vi "Generate Test Images.vi"() -> (0 "error out":errorcluster, 1 "queue out":refnum<queue>)   [LabVIEW 2018, in "Assembly Line Input.lvclass"]
doc: "Generate 50 test images of each type of board, with randomized failures."
uses:
  Assembly Line Input.lvclass
  Common/Board Type Enum.ctl
  Common/Board Image.ctl
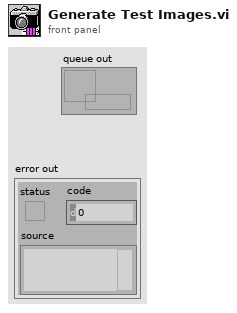
[diagram p1: front panel]
types:
  T1 = typedef "Board Type Enum.ctl" = enum16{"Basic DAQ Board", "Elite DAQ Board", "GPIB Board"}
  T2 = typedef "Board Image.ctl" = picture
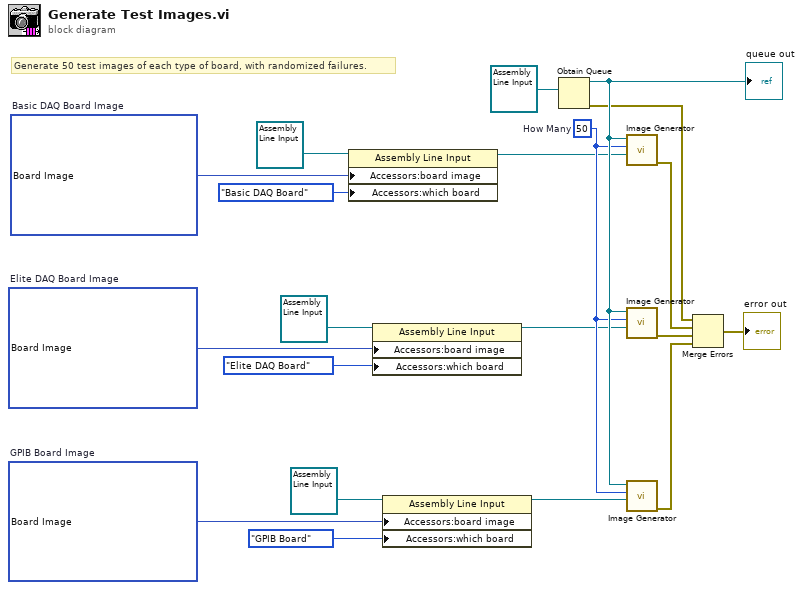
[diagram p0: block diagram]
diagram:
  w1 = T2 bytes[67710]  # GPIB Board Image
  w6 = T2 bytes[67710]  # Elite DAQ Board Image
  w11 = T2 bytes[67710]  # Basic DAQ Board Image
  w19 = 50  # How Many
  # "Generate 50 test images of each type of board, with randomized failures."
  n1 = property class="Assembly Line Input"(reference=refnum<class "Assembly Line Input.lvclass"> refnum ("Assembly Line Input"), "Accessors:board image"=w11, "Accessors:which board"=Board_Type_Enum."Basic DAQ Board" ("which board")) -> (reference out=w9:refnum<class "Assembly Line Input.lvclass">)  [unwired: 1 in, 1 out]
  n2 = property class="Assembly Line Input"(reference=refnum<class "Assembly Line Input.lvclass"> refnum ("Assembly Line Input"), "Accessors:board image"=w6, "Accessors:which board"=Board_Type_Enum."Elite DAQ Board" ("which board")) -> (reference out=w4:refnum<class "Assembly Line Input.lvclass">)  [unwired: 1 in, 1 out]
  n3 = property class="Assembly Line Input"(reference=refnum<class "Assembly Line Input.lvclass"> refnum ("Assembly Line Input"), "Accessors:board image"=w1, "Accessors:which board"=Board_Type_Enum."GPIB Board" ("which board")) -> (reference out=w2:refnum<class "Assembly Line Input.lvclass">)  [unwired: 1 in, 1 out]
  n4 = Obtain Queue(element data type=refnum<class "Assembly Line Input.lvclass"> refnum ("Assembly Line Input")) -> (queue out=w20:refnum<queue>, error out=w14:errorcluster)  [unwired: 4 in, 1 out]
  "queue out" <- w20
  n5 = call "Image Generator.vi"("Assembly Line Input"=w9, "how many"=w19, "Queue in"=w20) -> ("error out"=w18:errorcluster)  [unwired: 8 in]
  n6 = call "Image Generator.vi"("Assembly Line Input"=w4, "how many"=w19, "Queue in"=w20) -> ("error out"=w17:errorcluster)  [unwired: 8 in]
  n7 = call "Image Generator.vi"("Assembly Line Input"=w2, "how many"=w19, "Queue in"=w20) -> ("error out"=w16:errorcluster)  [unwired: 8 in]
  n8 = Merge Errors(w14, w18, w17, w16) -> (→"error out":errorcluster)
